vi "Boundary Layer Lab.vi"() -> ()   [LabVIEW 2022 SP3]
uses:
  Anemometry/Anemometry Sub Vis/Controls/User_Specific_mode.ctl
  Anemometry/Anemometry Sub Vis/Gen Trav/Trav_mode.ctl
  Anemometry/Anemometry Sub Vis/Controls/Tunnel_Coordinates.ctl
  Anemometry/Anemometry Sub Vis/Controls/Save_Data.ctl
  Anemometry/Anemometry Sub Vis/Gen Trav/Spacing.ctl
  Anemometry/Anemometry Sub Vis/Controls/Multi_run_mode.ctl
  Anemometry/Anemometry Sub Vis/Gen Trav/Traverse_cluster.ctl
  ADAM Client/Sub VIs/ADAM Controls/Tunnel_speed_mode.ctl
panel:
  in  "2nd Profile active":bool
  in  "Seconds to Settle":u32=3
  out "Profile 2":cluster{dbl[], dbl[]}
  out "Profile1":cluster{dbl[], dbl[]}
  out "Currently on":enum16{"Profile 1", "Profile 2"}(ring)=enum."Profile 2"
  in  "Delta (mm) Profile 2":dbl=6.7 min=0.0 max=10.0 step=0.05 format="%.2f"
  in  "X (mm) Profile 2":sgl=550.0
  in  "X (mm) Profile 1":sgl=300.0
  in  "Offset (mm)":dbl step=0.05 format="%.2f"
  out "Blasius":cluster{"U/Uref":dbl[], "Z/Delta":dbl[]}={"U/Uref"=[0.0, 0.066, 0.133, 0.199, 0.265, 0.33, 0.394, 0.517, 0.63, 0.729, 0.812, 0.876, 0.923, 0.956, 0.992, 0.999, 1.0], "Z/Delta"=[0.0, 0.04, 0.08, 0.12, 0.16, 0.2, 0.24, 0.32, 0.4, 0.48, 0.56, 0.64, 0.72, 0.8, 1.0, 1.2, 1.5]}
  out "Comparison to Blasius":cluster{"U/Uref":dbl[], "Z/Delta":dbl[]}[](graph)
  in  "Delta (mm) Profile 1":dbl=6.7 min=0.0 max=10.0 step=0.05 format="%.2f"
  in  "Freestream Velocity (m/s)":dbl=7.23
  in  "Tunnel Speed":dbl=7.0
  in  "End Position (mm)":sgl=12.0
  in  "Zero Pressure Transducers":bool
  in  "Take Traverse Profiles":bool
  out "Velocity Profile":cluster{dbl[], dbl[]}[](graph)
  in  "stop":bool=TRUE
  in  "Number of Points":i32=12
  in  "Start Position (mm)":sgl=0.53
  in  "Averaging time (Sec)":dbl=5.0
  in  "Filename":path=path "\\\\surrey.ac.uk\\personal/HS103/m13602/Documents/Boundary Layer Lab/test6.xls"
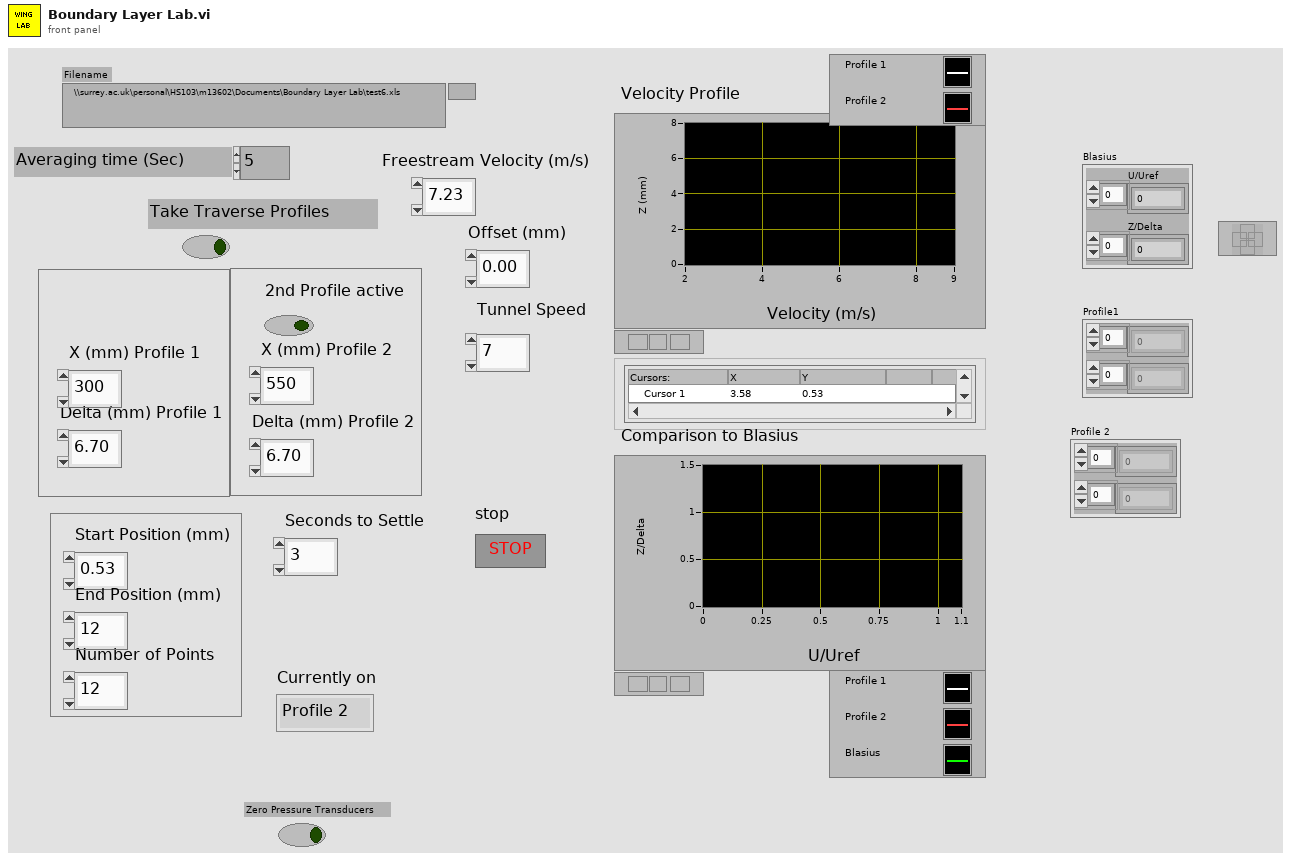
[diagram p1: front panel]
types:
  T1 = enum8{"Enabled", "Disabled", "Disabled and Grayed Out"}
  T2 = typedef "Tunnel_speed_mode.ctl" = enum16{"Set Speed", "Set Speed then wait", "Is tunnel speed allowable?"}
  T3 = typedef "User_Specific_mode.ctl" = enum16{"Check VI only", "Run VI"}
  T4 = typedef "Traverse_cluster.ctl" = cluster{"Start X":sgl, "Start Y":sgl, "Start Z":sgl, "End X":sgl, "End Y":sgl, "End Z":sgl, "nPoints":i32, "Spacing":T5, "Filename":path, "Tunnel Speed":dbl, "Averaging time (mins)":dbl, "Extra Commands":string, "Carrier_1 Q (l/min)":dbl, "Carrier_2 Q (l/min)":dbl, "Trace Gas Concentration (%)":dbl, "Specific Arguments":string, "Comments":string, "Row No":i32, "Row Type Selector":T6, "EstCompl":string, "Row Duration (mins)":dbl, "nValidPoints":i32, "Meas Setup File":string}
  T5 = typedef "Spacing.ctl" = enum16{"Linear", "Log", "Gauss", "Specified", "N/A"}
  T6 = typedef "Multi_run_mode.ctl" = enum16{"Move Traverse Only", "Set Tunnel Speed Only", "Set Source Only", "Set Measurement Conditions", "Single Measurement", "Vertical Profile", "Lateral Profile", "Longitudinal Profile", "Multi-Axis Profile", "Explore Volume", "Auto Calibrate", "Meas Fast FID Bkgnd", "Check Beam Power", "Scanning Valve Measurement", "Run VI Named:", "Set ADAM Ch", "Wait (minutes)", "Send Message", "Synchronize With:", "Fall Back to this Row", "Turn Off Row Repeating", "Traverse 3D Volume", "Blank Row", "Jump to Fall Back Row"}
  T7 = typedef "Tunnel_Coordinates.ctl" = enum16{"Work in Tunnel Coordinates", "Work in Model Coordinates"}
  T8 = typedef "Trav_mode.ctl" = enum16{"Move traverse", "Read traverse position", "Teach Position"}
  T9 = typedef "Save_Data.ctl" = enum16{"Save No Data", "Save Data"}
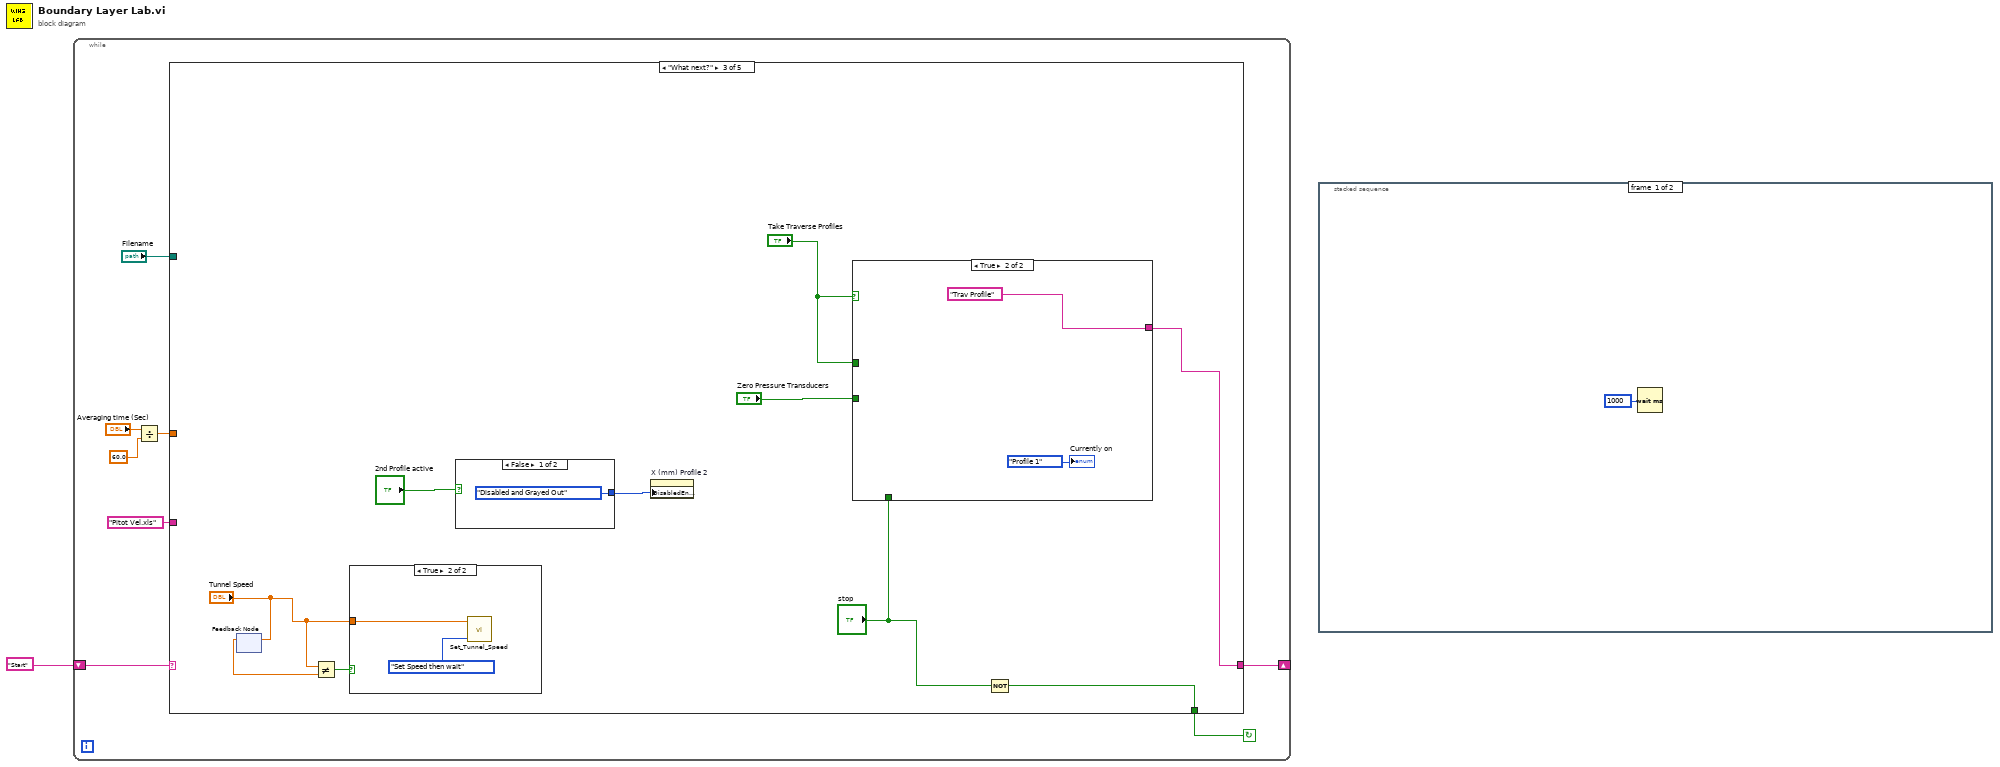
[diagram p0: block diagram]
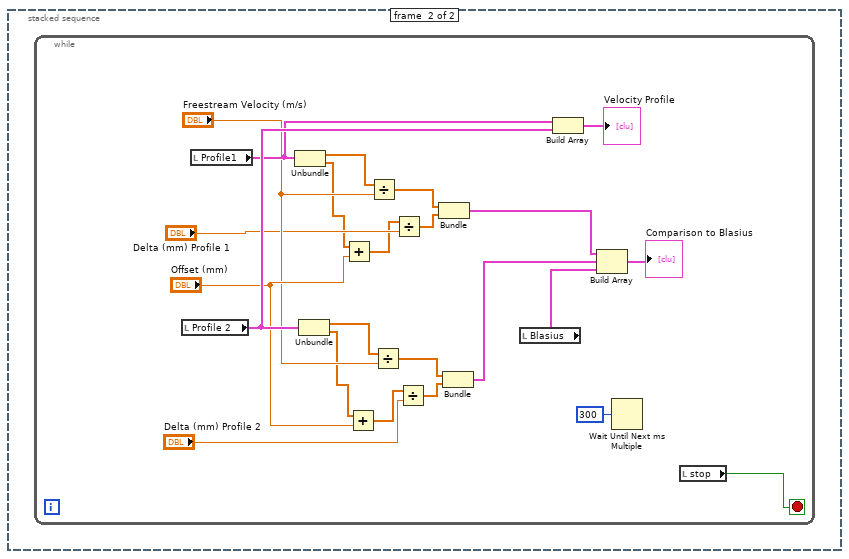
[diagram p2: hidden frame]
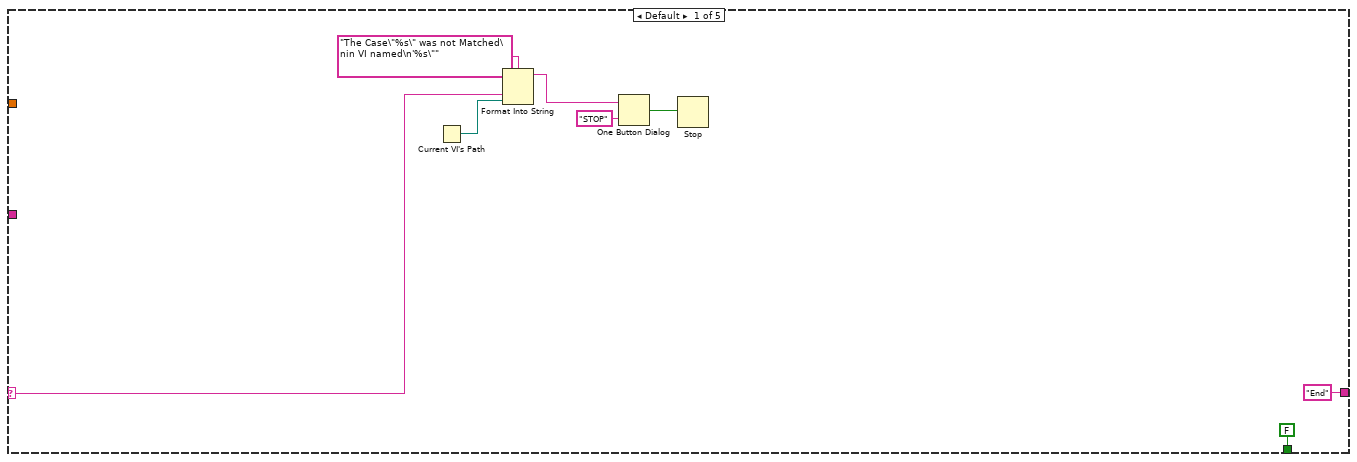
[diagram p3: hidden frame]
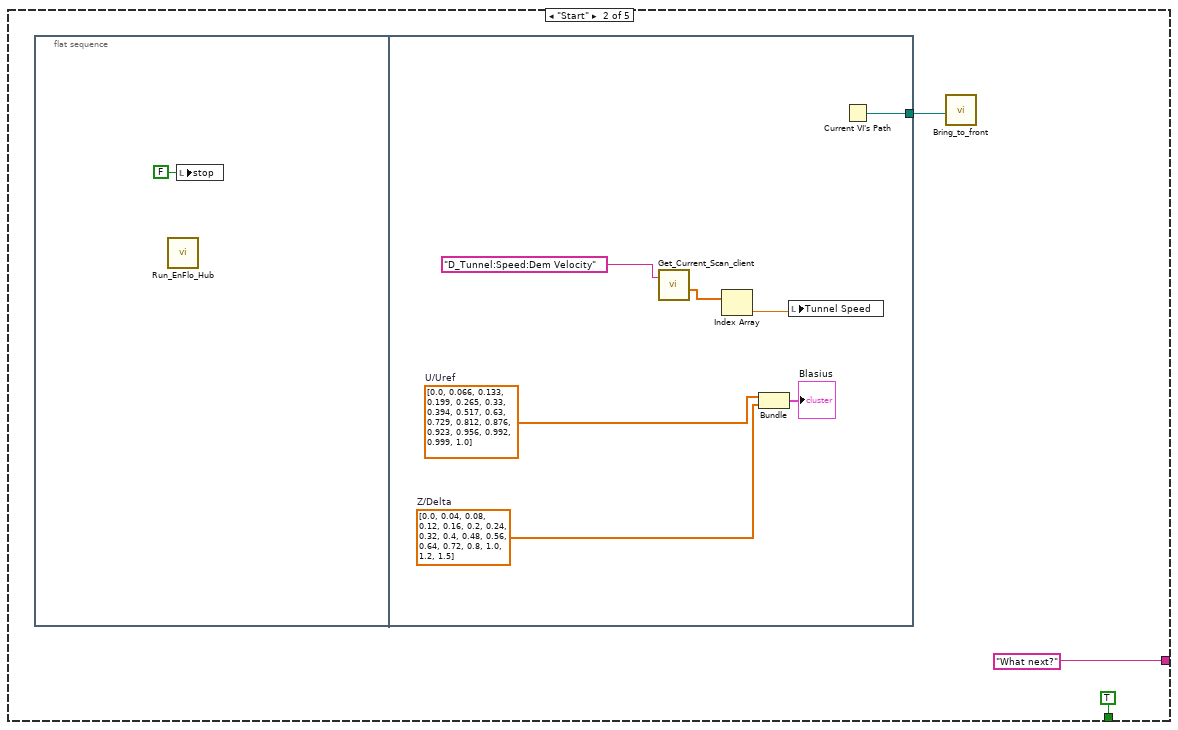
[diagram p4: hidden frame]
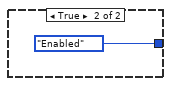
[diagram p5: hidden frame]
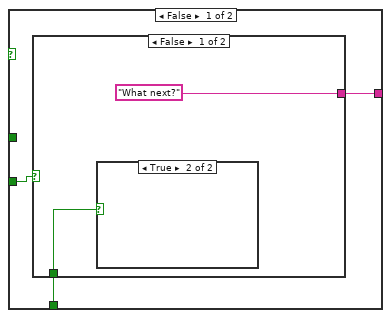
[diagram p6: hidden frame]
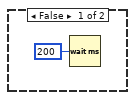
[diagram p7: hidden frame]
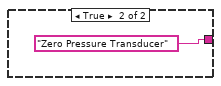
[diagram p8: hidden frame]
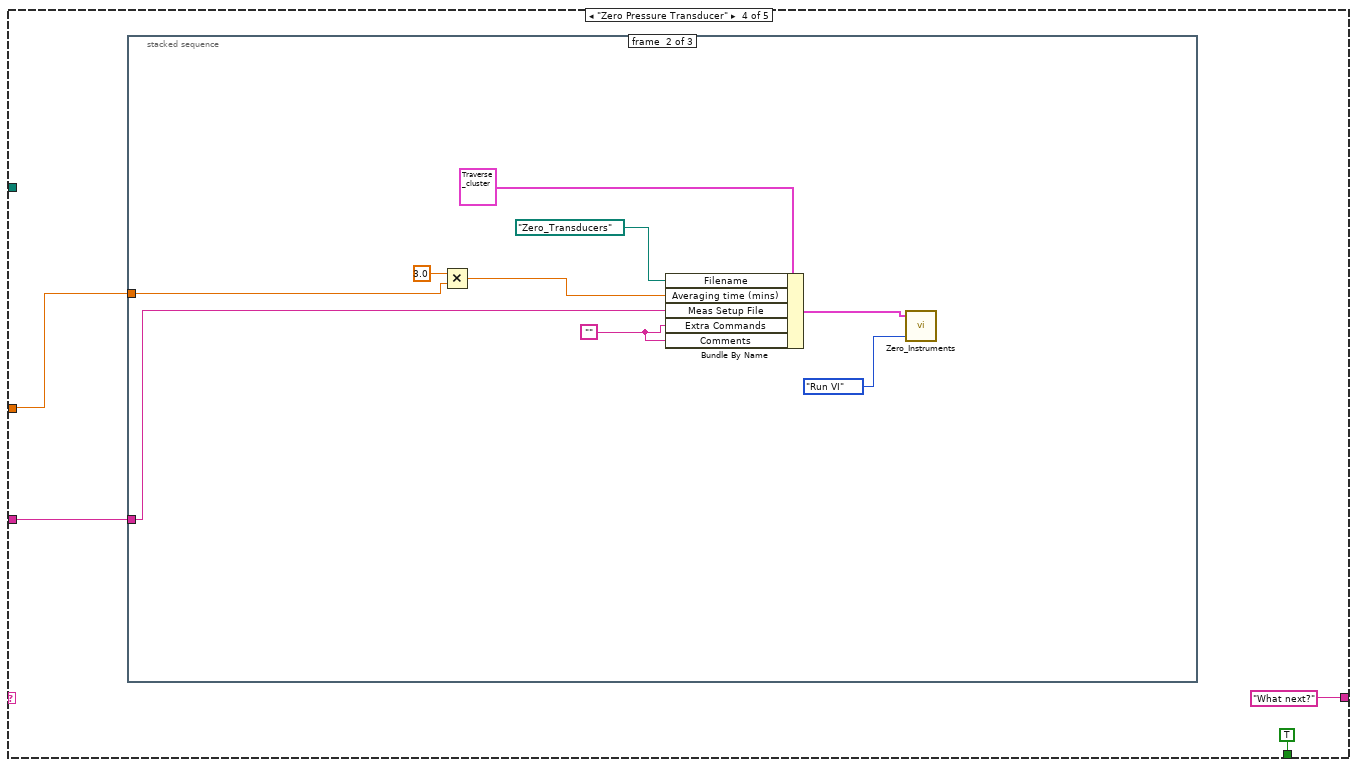
[diagram p10: hidden frame]
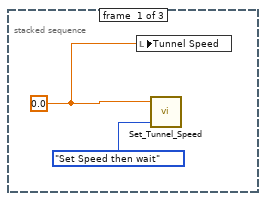
[diagram p11: hidden frame]
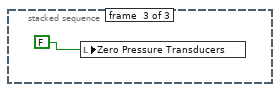
[diagram p12: hidden frame]
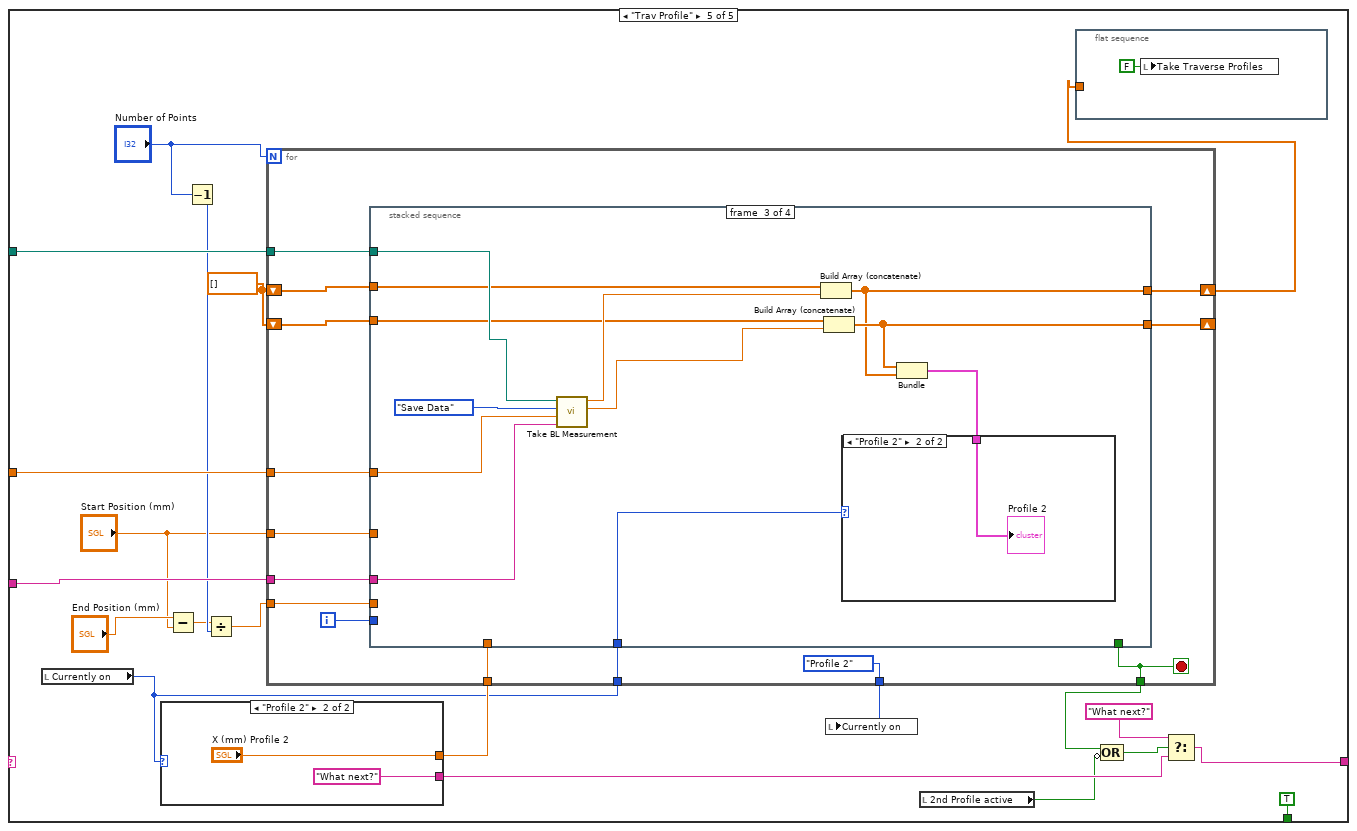
[diagram p13: hidden frame]
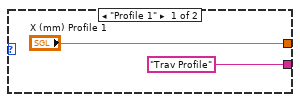
[diagram p14: hidden frame]
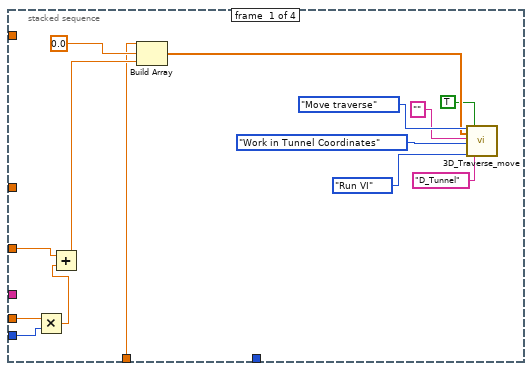
[diagram p15: hidden frame]
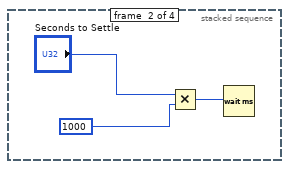
[diagram p16: hidden frame]
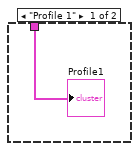
[diagram p17: hidden frame]
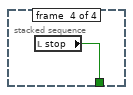
[diagram p18: hidden frame]
diagram:
  n1 = while {
    shift-right: [w3] -> _
    shift-left: "Start" -> [w8]
    stop <- w9 continue-if-true
    n2 = Divide(x="Averaging time (Sec)", y=60.0) -> (x/y=w4:dbl)
    n3 = case shown="\"What next?\"" w8 {
      selector: w8 -> [w12 _ _ _ _]
      tunnel: [FALSE ("Stop Button") TRUE ("Stop Button") w38 TRUE ("Stop Button") TRUE ("Stop Button")] -> w9
      tunnel: "Filename" -> [_ _ _ _ w88]
      tunnel: w4 -> [_ _ _ w52 w87]
      tunnel: ["End" "What next?" w37 "What next?" w71] -> w3
      tunnel: "Pitot Vel.xls" ("Setup filename") -> [_ _ _ w55 w84]
      frame Default {
        n4 = Current VI's Path() -> (path=w17:path)
        n5 = Format Into String(format string="The Case\"%s\" was not Matched\nin VI named\n'%s\"" ("Format String"), w12, w17) -> (resulting string=w14:string)  [unwired: 2 in, 1 out]
        n6 = One Button Dialog(message=w14, button name ("OK")="STOP") -> (true=w16:bool)
        n7 = Stop(stop? (T)=w16) -> ()
      }
      frame "Start" {
        n8 = flat-sequence {
          tunnel: [w28] -> w18
          frame #0 {
            n9 = call "Run_EnFlo_Hub.vi"() -> ()  [unwired: 7 in, 1 out]
            n10 = local write "stop"(FALSE ("stop")) -> ()
          }
          frame #1 {
            w24 = dbl[] [0.0, 0.066, 0.133, 0.199, 0.265, 0.33, 0.394, 0.517, 0.63, 0.729, 0.812, 0.876, 0.923, 0.956, 0.992, 0.999, 1.0]  # U/Uref
            w23 = dbl[] [0.0, 0.04, 0.08, 0.12, 0.16, 0.2, 0.24, 0.32, 0.4, 0.48, 0.56, 0.64, 0.72, 0.8, 1.0, 1.2, 1.5]  # Z/Delta
            n11 = call "Get_Current_Scan_client.vi"("singleChannel"="D_Tunnel:Speed:Dem Velocity") -> ("Numerical Values"=w26:dbl[])  [unwired: 1 in, 3 out]
            n12 = Index Array(array=w26) -> (element=w25:dbl)  [unwired: 1 in]
            n13 = Bundle("U/Uref"=w24, "Z/Delta"=w23) -> (→"Blasius":cluster{"U/Uref":dbl[], "Z/Delta":dbl[]})  [unwired: 1 in]
            n14 = local write "Tunnel Speed"(w25) -> ()
            n15 = Current VI's Path() -> (path=w28:path)
          }
        }
        n16 = call "Bring_to_front.vi"("path"=w18) -> ()
      }
      frame "What next?" {
        n17 = feedback-in #1("Tunnel Speed") -> ()
        n18 = feedback #1() -> (w34:dbl)  [unwired: 1 in]
        n19 = Not Equal?(x="Tunnel Speed", y=w34) -> (x != y?=w33:bool)
        n20 = case shown="True" w33 {
          tunnel: "Tunnel Speed" -> [_ w51]
          frame False {
          }
          frame True {
            n21 = call "Set_Tunnel_Speed.vi"("Mode"=Tunnel_speed_mode."Set Speed then wait", "Tunnel Velocity m/s"=w51) -> ()  [unwired: 2 in, 2 out]
          }
        }
        n22 = case shown="False" "2nd Profile active" {
          tunnel: [T1."Disabled and Grayed Out" ("Disabled") T1."Enabled" ("Disabled")] -> w30
          frame False {
          }
          frame True {
          }
        }
        n23 = property on="X (mm) Profile 2" class="DigNum (strict)"("DisabledEnum"=w30) -> ()  [unwired: 2 in, 2 out]
        n24 = case shown="True" "Take Traverse Profiles" {
          tunnel: "Take Traverse Profiles" -> [_ _]
          tunnel: [w43 "Trav Profile"] -> w37
          tunnel: "stop" -> [w42 _]
          tunnel: "Zero Pressure Transducers" -> [w41 _]
          frame False {
            n25 = case shown="False" w41 {
              tunnel: ["What next?" "Zero Pressure Transducer"] -> w43
              tunnel: w42 -> [w44 _]
              frame False {
                n26 = case shown="True" w44 {
                  frame False {
                    n27 = Wait (ms)(milliseconds to wait=u32 200) -> ()  [unwired: 1 out]
                  }
                  frame True {
                  }
                }
              }
              frame True {
              }
            }
          }
          frame True {
            "Currently on" <- enum16{"Profile 1", "Profile 2"}."Profile 1" ("Profile")
          }
        }
        n28 = Not(x="stop") -> (.not. x?=w38:bool)
      }
      frame "Zero Pressure Transducer" {
        n29 = stacked-sequence {
          tunnel: w55 -> [_ w64 _]
          tunnel: w52 -> [_ w60 _]
          frame #0 {
            w56 = 0.0 ("Tunnel Velocity m/s")
            n30 = local write "Tunnel Speed"(w56) -> ()
            n31 = call "Set_Tunnel_Speed.vi"("Mode"=Tunnel_speed_mode."Set Speed then wait", "Tunnel Velocity m/s"=w56) -> ()  [unwired: 2 in, 2 out]
          }
          frame #1 {
            w61 = ""
            n32 = Multiply(x=3.0, y=w60) -> (x*y=w59:dbl)
            n33 = Bundle By Name(cluster=T4 {"Start X"=0.0, "Start Y"=0.0, "Start Z"=0.0, "End X"=0.0, "End Y"=0.0, "End Z"=0.0, "nPoints"=0, "Spacing"=enum."Linear", "Filename"=path "", "Tunnel Speed"=0.0, "Averaging time (mins)"=0.0, "Extra Commands"="", "Carrier_1 Q (l/min)"=0.0, "Carrier_2 Q (l/min)"=0.0, "Trace Gas Concentration (%)"=0.0, "Specific Arguments"="", "Comments"="", "Row No"=0, "Row Type Selector"=enum."Move Traverse Only", "EstCompl"="", "Row Duration (mins)"=0.0, "nValidPoints"=0, "Meas Setup File"=""} ("Traverse line In"), "Filename"=path "Zero_Transducers", "Averaging time (mins)"=w59, "Meas Setup File"=w64, "Extra Commands"=w61, "Comments"=w61) -> (w63:T4)
            n34 = call "Zero_Instruments.vi"("Mode"=User_Specific_mode."Run VI", "Traverse line In"=w63) -> ()  [unwired: 1 in, 3 out]
          }
          frame #2 {
            n35 = local write "Zero Pressure Transducers"(FALSE ("Take Traverse Profile")) -> ()
          }
        }
      }
      frame "Trav Profile" {
        w86 = dbl[] []
        n36 = local read "Currently on"() -> (w75:enum16{"Profile 1", "Profile 2"})
        n37 = case shown="\"Profile 2\"" w75 {
          tunnel: ["X (mm) Profile 1" "X (mm) Profile 2"] -> w76
          tunnel: ["Trav Profile" "What next?"] -> w72
          frame "Profile 1" {
          }
          frame "Profile 2" {
          }
        }
        n38 = Subtract(x="End Position (mm)", y="Start Position (mm)") -> (x-y=w80:sgl)
        n39 = Decrement(x="Number of Points") -> (x-1=w81:i32)
        n40 = Divide(x=w80, y=w81) -> (x/y=w77:sgl)
        n41 = for {
          N: "Number of Points" -> [_]
          tunnel: w88 -> [w107]
          tunnel: w87 -> [w106]
          tunnel: w77 -> [w104]
          tunnel: "Start Position (mm)" -> [w103]
          shift-right: [w101] -> w83
          shift-left: w86 -> [w102]
          shift-right: [w99] -> _
          shift-left: w86 -> [w100]
          tunnel: w84 -> [w98]
          tunnel: w76 -> [w97]
          tunnel: w75 -> [w96]
          tunnel: [enum16{"Profile 1", "Profile 2"}."Profile 2" ("Profile")] -> w74
          tunnel: [w94] -> w69
          i -> [w105]
          stop <- w94 stop-if-true
          n42 = stacked-sequence {
            tunnel: w107 -> [_ _ w136 _]
            tunnel: w106 -> [_ _ w134 _]
            tunnel: w105 -> [w111 _ _ _]
            tunnel: w104 -> [w116 _ _ _]
            tunnel: w103 -> [w114 _ _ _]
            tunnel: w102 -> [_ _ w133 _]
            tunnel: [_ _ w127 _] -> w101
            tunnel: w100 -> [_ _ w130 _]
            tunnel: [_ _ w128 _] -> w99
            tunnel: w98 -> [_ _ w129 _]
            tunnel: [_ _ _ w139] -> w94
            tunnel: w97 -> [w108 _ _ _]
            tunnel: w96 -> [_ _ w125 _]
            frame #0 {
              n43 = Multiply(x=w116, y=w111) -> (x*y=w115:sgl)
              n44 = Add(x=w114, y=w115) -> (x+y=w113:sgl)
              n45 = Build Array(w108, sgl 0.0 ("element"), w113) -> (w112:sgl[])
              n46 = call "3D_Traverse_move.vi"("Mode"=Trav_mode."Move traverse", "Position"=w112, "Extra command String"="", "Work in Tunnel Coordinates"=Tunnel_Coordinates."Work in Tunnel Coordinates", "Simulate/Run"=User_Specific_mode."Run VI", "Route Checking?"=TRUE, "Traverse name"="D_Tunnel") -> ()  [unwired: 9 in, 4 out]
            }
            frame #1 {
              n47 = Multiply(x="Seconds to Settle", y=u32 1000 ("millisecond timer value")) -> (x*y=w123:u32)
              n48 = Wait (ms)(milliseconds to wait=w123) -> ()  [unwired: 1 out]
            }
            frame #2 {
              n49 = call "Take BL Measurement.vi"("Setup filename"=w129, "Averaging time (min)"=w134, "File"=Save_Data."Save Data", "Filename"=w136) -> ("U Trav"=w131:dbl, "Z"=w132:dbl)  [unwired: 5 in, 1 out]
              n50 = Build Array (concatenate)(w133, w132) -> (w127:dbl[])
              n51 = Build Array (concatenate)(w130, w131) -> (w128:dbl[])
              n52 = Bundle(w128, w127) -> (w126:cluster{dbl[], dbl[]})  [unwired: 1 in]
              n53 = case shown="\"Profile 2\"" w125 {
                tunnel: w126 -> [w137 w138]
                frame "Profile 1" {
                  "Profile1" <- w137
                }
                frame "Profile 2" {
                  "Profile 2" <- w138
                }
              }
            }
            frame #3 {
              n54 = local read "stop"() -> (w139:bool)
            }
          }
        }
        n55 = local write "Currently on"(w74) -> ()
        n56 = local read "2nd Profile active"() -> (w70:bool)
        n57 = flat-sequence {
          tunnel: w83 -> [_]
          frame #0 {
            n58 = local write "Take Traverse Profiles"(FALSE ("Take Traverse Profile")) -> ()
          }
        }
        n59 = Compound Arithmetic op=OR(w69, invert w70) -> (w68:bool)
        n60 = Select(t="What next?", s=w68, f=w72) -> (s? t:f=w71:string)
      }
    }
  }
  n61 = stacked-sequence {
    frame #0 {
      n62 = Wait (ms)(milliseconds to wait=u32 1000) -> ()  [unwired: 1 out]
    }
    frame #1 {
      n63 = while {
        stop <- w142 stop-if-true
        n64 = local read "Profile 2"() -> (w163:cluster{dbl[], dbl[]})
        n65 = local read "Profile1"() -> (w161:cluster{dbl[], dbl[]})
        n66 = Unbundle(w161) -> (w143:dbl[], w146:dbl[])
        n67 = Unbundle(w163) -> (w153:dbl[], w150:dbl[])
        n68 = Add(x=w146, y="Offset (mm)") -> (x+y=w147:dbl[])
        n69 = Add(x=w150, y="Offset (mm)") -> (x+y=w149:dbl[])
        n70 = Divide(x=w143, y="Freestream Velocity (m/s)") -> (x/y=w144:dbl[])
        n71 = Divide(x=w153, y="Freestream Velocity (m/s)") -> (x/y=w152:dbl[])
        n72 = Divide(x=w147, y="Delta (mm) Profile 1") -> (x/y=w145:dbl[])
        n73 = Divide(x=w149, y="Delta (mm) Profile 2") -> (x/y=w151:dbl[])
        n74 = Bundle(w144, w145) -> (w157:cluster{dbl[], dbl[]})  [unwired: 1 in]
        n75 = Bundle(w152, w151) -> (w158:cluster{dbl[], dbl[]})  [unwired: 1 in]
        n76 = local read "Blasius"() -> (w159:cluster{"U/Uref":dbl[], "Z/Delta":dbl[]})
        n77 = Build Array(w161, w163) -> (→"Velocity Profile":cluster{dbl[], dbl[]}[])
        n78 = Build Array(w157, w158, w159) -> (→"Comparison to Blasius":cluster{"U/Uref":dbl[], "Z/Delta":dbl[]}[])
        n79 = Wait Until Next ms Multiple(millisecond multiple=u32 300) -> ()  [unwired: 1 out]
        n80 = local read "stop"() -> (w142:bool)
      }
    }
  }
